vi "BG_Remove.vi"(1 "BG Data":dbl[][][](array[numeric]), 2 "Data IN":dbl[][][](array[numeric])) -> (0 "Data OUT":dbl[][][](array[numeric]))   [LabVIEW 2016]
panel:
  out "3":dbl[](graph)
  out "2":dbl[](graph)
  out "1":dbl[](graph)
  out "BG Array":dbl[](array[numeric])
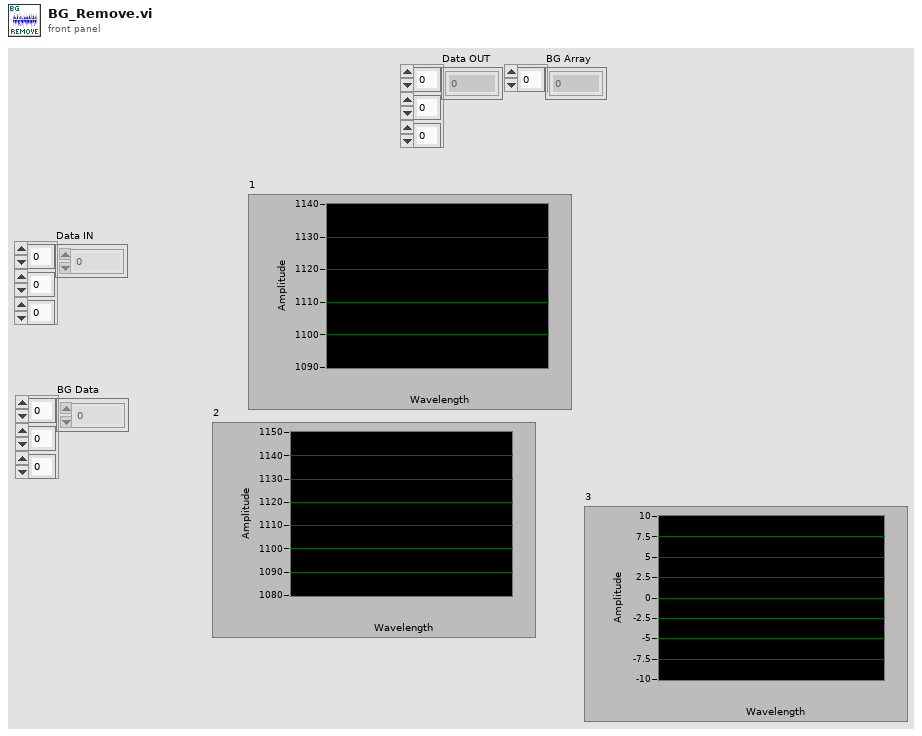
[diagram p1: front panel]
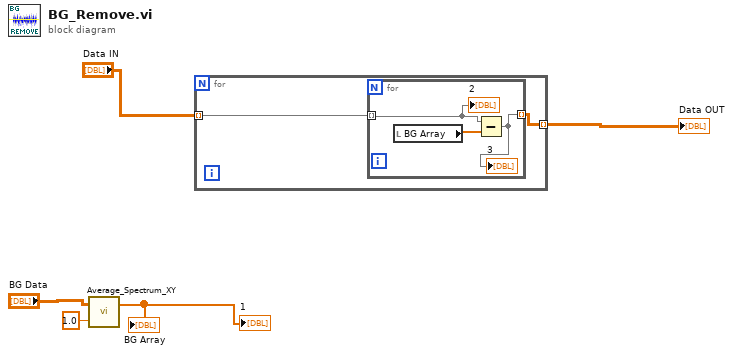
[diagram p0: block diagram]
diagram:
  n1 = call "Average_Spectrum_XY.vi"("Multiplyer"=1.0, "Array IN 3D"="BG Data") -> ("Array Out 1D"=→"BG Array" →"1":dbl[])  [unwired: 1 out]
  n2 = for {
    tunnel: "Data IN" -> [w7] mode=indexing
    tunnel: [w6] -> w1 mode=indexing
    n3 = for {
      tunnel: [w8] -> w6 mode=indexing
      tunnel: w7 -> [w9] mode=indexing
      n4 = local read "BG Array"() -> (w10:dbl[])
      n5 = Subtract(x=w9, y=w10) -> (x-y=w8:dbl[])
      "3" <- w8
      "2" <- w9
    }
  }
  "Data OUT" <- w1
